vi "Vision Processing.vi"(4 "error in (no error)":errorcluster, 6 "CameraDevRef":T1) -> ()   [LabVIEW 2011]
uses:
  <vilib>/Rock Robotics/WPI/Camera/WPI_CameraDevRef.ctl
  Robot Global Data.vi
  <vilib>/vision/NI_Vision_Development_Module.lvlib
panel:
  in  "AntiDrift":dbl=-0.065
  in  "Y AbsolVal Difference":dbl=0.25
  in  "Default Shooter Speed Dump":dbl=0.4
  in  "Scale":dbl=0.85
  in  "Minimum Power":dbl=0.22
  out "Aspect Ratio":dbl[](array[numeric])
  out "Offset":dbl
  out "Raw Turret":dbl
  out "Target X Coord":dbl
  out "Target Distance":dbl
  out "Distance Array":dbl[](array[numeric])
  in  "Dead Band":dbl=0.09
  out "Number of Rectangles Visible":dbl
  out "Y Position Array":dbl[](array[numeric])
  out "X Position Array":dbl[](array[numeric])
  in  "View":bool
  out "Target Info":T2(array[cluster])
  in  "Area Size Limit":i32=444
  in  "Particle Count Limit":i32=8
  in  "Score Limits":T3={"Rect Coverage"=76.0, "Aspect Ratio"=40.0, "X Edge Strength"=40.0, "Y Edge Strength"=60.0}
  in  "Processing":enum32{"Color", "Intensity", "Intensity Open"}(tab)=enum."Intensity"
  in  "Luminance":i32=255
  in  "Saturation":i32=255
  in  "Hue":i32(knob)=65 scale=0.0..255.0
  in  "Margins":cluster{"Hue":i32, "Sat":i32, "Lum":i32}={"Hue"=20, "Sat"=27, "Lum"=30} {"Sat" scale=0.0..40.0; "Lum" scale=0.0..40.0; "Hue" scale=0.0..40.0}
  in  "Range":cluster{"Lower value":sgl, "Upper value":sgl}={"Lower value"=151.52174, "Upper value"=255.0} {"Lower value" scale=0.0..255.0; "Upper value" scale=0.0..255.0}
  in  "Range":cluster{"Lower value":sgl, "Upper value":sgl}={"Lower value"=123.804344, "Upper value"=255.0} {"Lower value" scale=0.0..255.0; "Upper value" scale=0.0..255.0}
  in  "View":bool
  out "Processed Image":T4(plugin-control)
  out "Original Image":T4(plugin-control)
  # "Instructions:\nProcessing the reflective tape that is illuminated by a ring light can be based\non color or light intensity.\nParticles within the image are scored by rectangle coverage, aspect ratio, and\nfor being hollow with a bold edge. A particle is considered a target if all scores\nare above the score limits. Particles can be annotated -- surrounded by\na rectangle and scores drawn to the left .\nTo control the number of particles being scored, use the count limit and the size\nlimit."
  # "(in)"
  # "To debug, Enable using the View button.\nFor color processing, you can click in the image to select the color for processing."
  # "Enable by clicking the View button.\nGreen scores are above the limit, orange are below. Inner/outer rect\nindicates all passed."
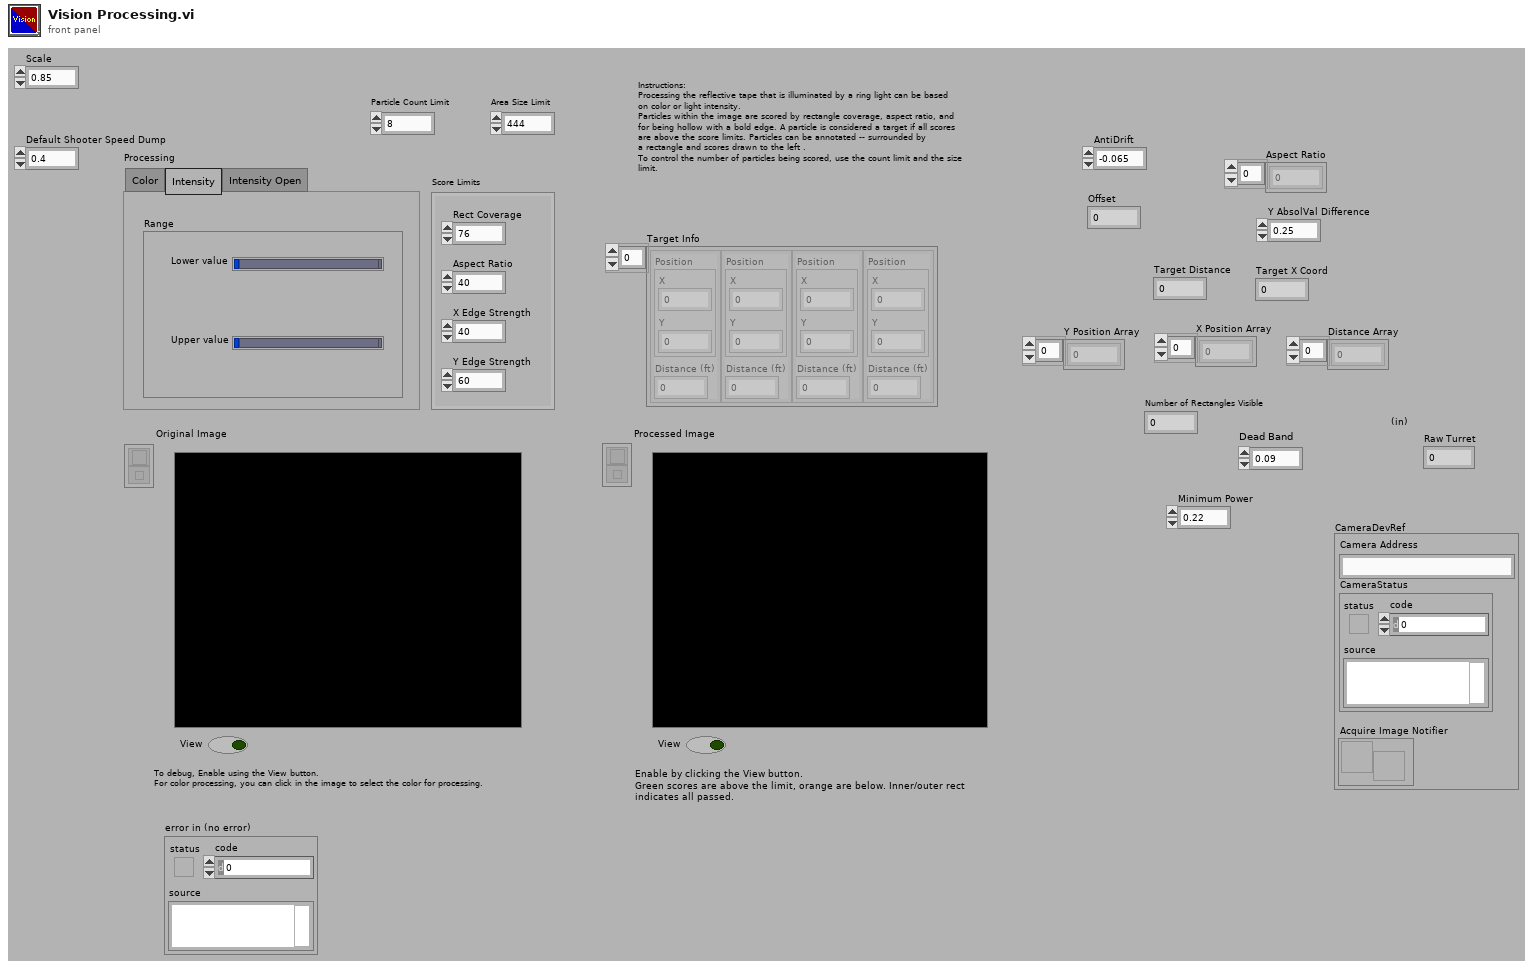
[diagram p1: front panel]
types:
  T1 = typedef "WPI_CameraDevRef.ctl" = cluster{"Camera Address":string, "CameraStatus":errorcluster, "Acquire Image Notifier":refnum<notifier>}
  T2 = cluster{"Position":cluster{"X":dbl, "Y":dbl}, "Distance (ft)":dbl}[]
  T3 = cluster{"Rect Coverage":dbl, "Aspect Ratio":dbl, "X Edge Strength":dbl, "Y Edge Strength":dbl}
  T4 = typedef "IMAQ Image.ctl" = refnum<image>
  T5 = typedef "Image Type" = u32
  T6 = enum32{"AutoM", "Close", "Dilate", "Erode", "Gradient", "Gradient out", "Gradient in", "Hit miss", "Open", "PClose", "POpen", "Thick", "Thin"}
  T7 = typedef "WPI_CameraImageSize.ctl" = enum16{"640x480", "320x240", "160x120"}
  T8 = cluster{"fps":i32, "compression":i32, "Image Size":T7}
  T9 = cluster{cluster{"Left":dbl, "Top":dbl, "Right":dbl, "Bottom":dbl}, dbl[]}[]
  T10 = cluster{"Left":dbl, "Top":dbl, "Right":dbl, "Bottom":dbl}
  T11 = cluster{"Target Center (-1 to 1)":cluster{"X":dbl, "Y":dbl}, "Distance (ft)":dbl}
  T12 = cluster{"Target Center (-1 to 1)":cluster{"X":dbl, "Y":dbl}, "Distance (ft)":dbl}[]
  T13 = typedef "WPI_JoystickDevRef.ctl" = cluster{"Device":T14}
  T14 = typedef "WPI_JoystickDeviceEnum.ctl" = enum16{"USB 1", "USB 2", "USB 3", "USB 4", "Kinect 1", "Kinect 2"}
  T15 = typedef "WPI_JoystickButtonState.ctl" = cluster{"Button 1":bool, "Button 2":bool, "Button 3":bool, "Button 4":bool, "Button 5":bool, "Button 6":bool, "Button 7":bool, "Button 8":bool, "Button 9":bool, "Button 10":bool, "Button 11":bool, "Button 12":bool}
  T16 = cluster{"axis 1 (x)":dbl, "axis 2 (y)":dbl, "axis 3 (throttle)":dbl, "axis 4":dbl, "axis 5":dbl, "axis 6":dbl}
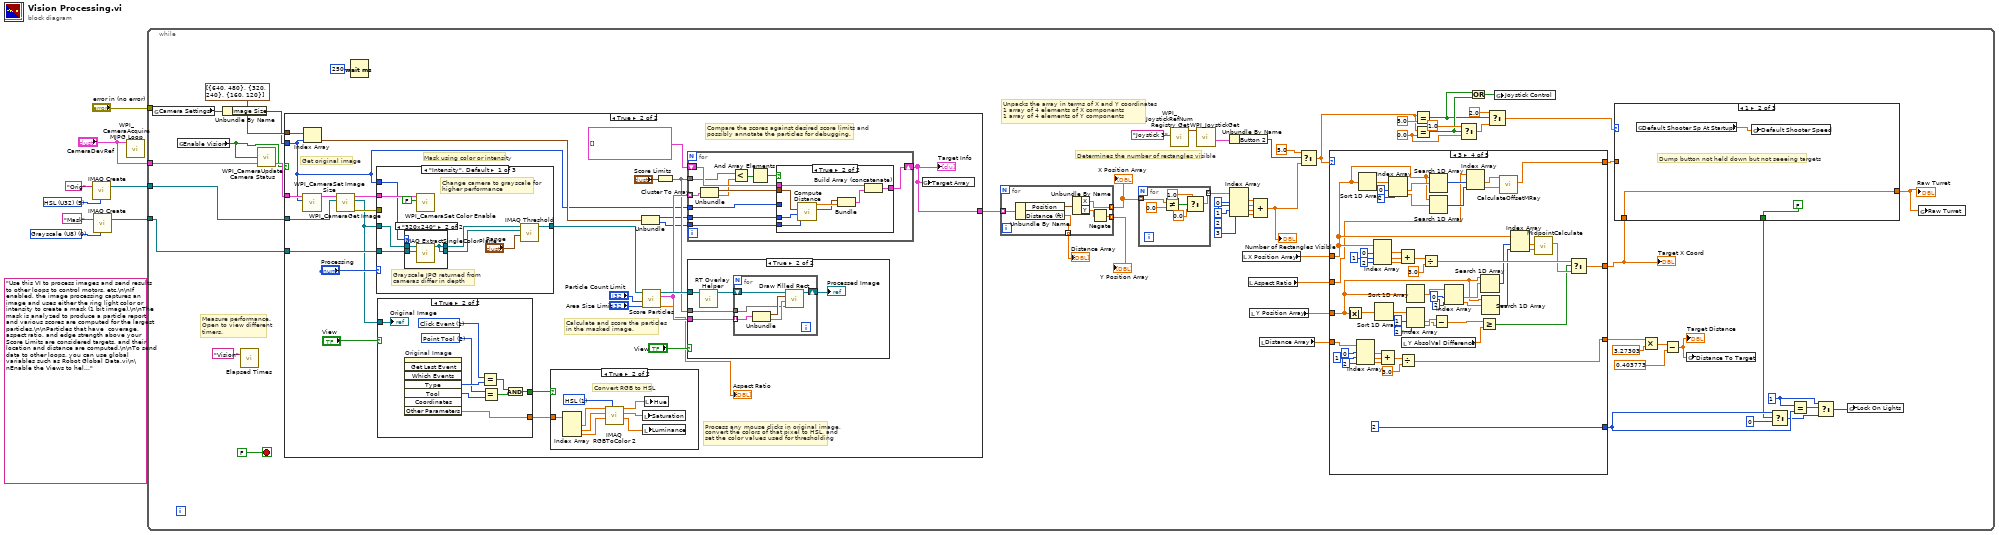
[diagram p0: block diagram]
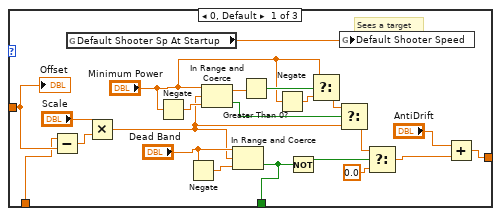
[diagram p2: hidden frame]
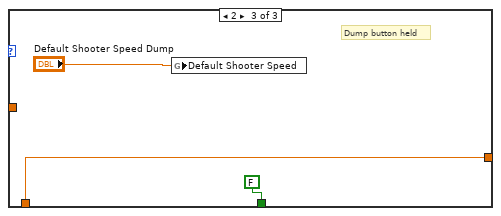
[diagram p3: hidden frame]
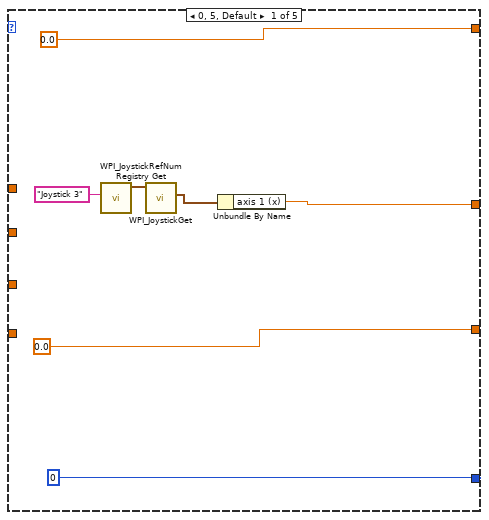
[diagram p4: hidden frame]
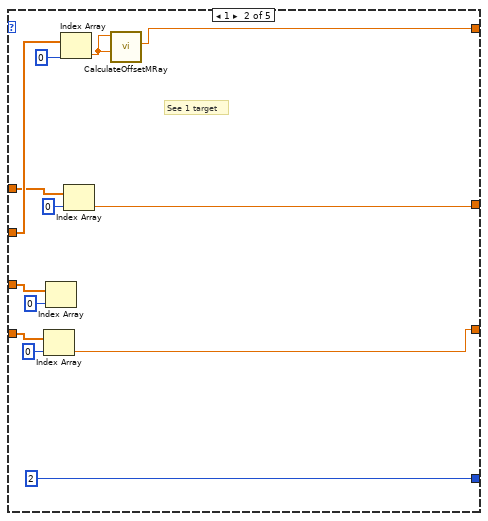
[diagram p5: hidden frame]
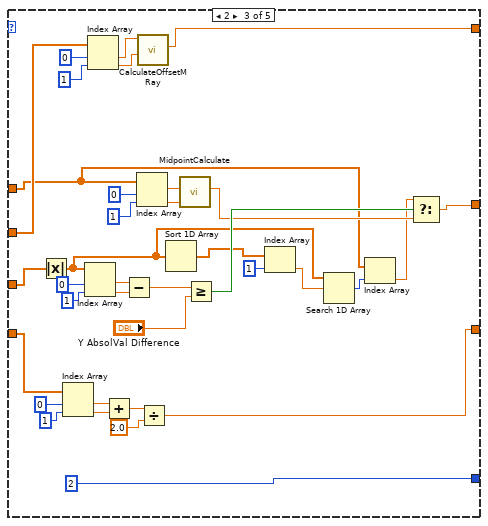
[diagram p6: hidden frame]
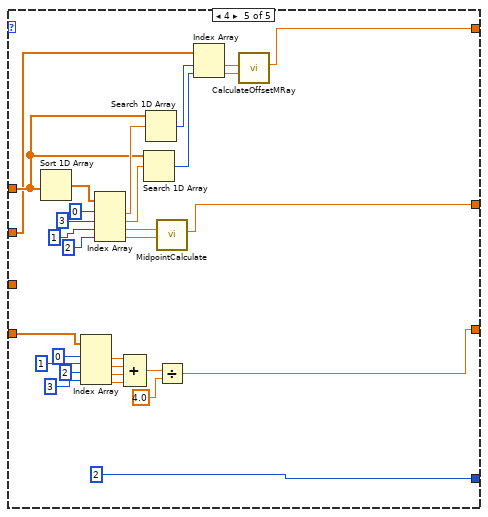
[diagram p7: hidden frame]
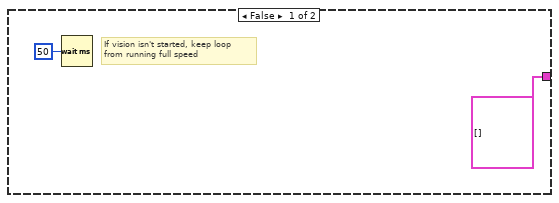
[diagram p8: hidden frame]
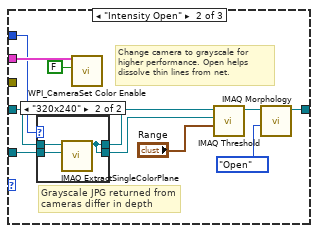
[diagram p11: hidden frame]
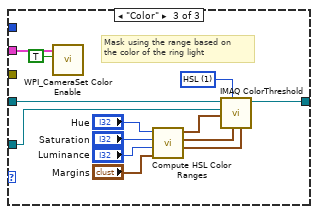
[diagram p13: hidden frame]
diagram:
  w3 = T5 0 items=["Grayscale (U8)", "Grayscale (I16)", "Grayscale (SGL)", "Complex (CSG)", "RGB (U32)", "HSL (U32)", "RGB (U64)", "Grayscale (U16)"] ("Image Type")
  (unwired) "Use this VI to process images and send results to other loops to control motors, etc.\n\nIf enabled, the image processing captures an image and uses either the ring light color or intensity to create a mask (1 bit image).\n\nThe mask is analyzed to produce a particle report and various scores are computed for the largest particles.\n\nParticles that have  coverage, aspect ratio, and edge strength above your Score Limits are considered targets, and their location and distance are computed.\n\nTo send data to other loops, you can use global variables such as Robot Global Data.vi\n\nEnable the Views to help debug color settings. Disable the View to speed up processing."
  w7 = T5 5 items=["Grayscale (U8)", "Grayscale (I16)", "Grayscale (SGL)", "Complex (CSG)", "RGB (U32)", "HSL (U32)", "RGB (U64)", "Grayscale (U16)"] ("Image Type")
  n1 = call "IMAQ Create"("Image Name"="Orig", "Image Type"=w7) -> ("New Image"=w6:T4)  [unwired: 2 in, 2 out]
  n2 = call "IMAQ Create"("Image Name"="Mask", "Image Type"=w3) -> ("New Image"=w1:T4)  [unwired: 2 in, 2 out]
  n3 = call <vilib>:"WPI_CameraAcquire MJPG Loop.vi"("CameraDevRef"="CameraDevRef") -> ()  [unwired: 11 in]
  n4 = while {
    tunnel: w6 -> [w66]
    tunnel: "CameraDevRef" -> [w65]
    tunnel: "error in (no error)" -> [_]
    tunnel: w1 -> [w61]
    stop <- FALSE stop-if-true
    w14 = 0.0 ("y")
    w31 = 1 ("y")
    # "Determines the number of rectangles visible"
    # "Unpacks the array in terms of X and Y coordinates\n1 array of 4 elements of X components\n1 array of 4 elements of Y components"
    # "Measure performance.\nOpen to view different\ntimers."
    n5 = global read "Robot Global Data.vi" "Camera Settings"() -> (w59:T8)
    n6 = global read "Robot Global Data.vi" "Enable Vision"() -> (w63:bool)
    n7 = Unbundle By Name(w59) -> ("Image Size"=w58:T7)
    n8 = call "Elapsed Times.vi"("Call Name"="Vision") -> ()  [unwired: 2 in, 1 out]
    n9 = call <vilib>:"WPI_CameraUpdate Camera Status.vi"("CameraDevRef In"=w65, "Enable Vision"=w63) -> ("CameraDevRef Out"=w64:T1)  [unwired: 3 in]
    n10 = case shown="True" w63 {
      tunnel: w66 -> [_ w266]
      tunnel: w64 -> [_ w262]
      tunnel: w61 -> [_ w253]
      tunnel: cluster{i32, i32}[] [{640, 480}, {320, 240}, {160, 120}] -> [_ w257]
      tunnel: w58 -> [_ w250]
      tunnel: [T2 [] w251] -> w57
      frame False {
        # "If vision isn't started, keep loop\nfrom running full speed"
        n11 = Wait (ms)(milliseconds to wait=u32 50) -> ()  [unwired: 1 out]
      }
      frame True {
        # "Compare the scores against desired score limits and\npossibly annotate the particles for debugging."
        # "Process any mouse clicks in original image,\nconvert the colors of that pixel to HSL, and\nset the color values used for thresholding"
        # "Calculate and score the particles\nin the masked image."
        # "Mask using color or intensity"
        # "Get original image"
        n12 = call <vilib>:"WPI_CameraSet Image Size.vi"("Image Size"=w250, "CameraDevRef"=w262) -> ("CameraDevRef Out"=w263:T1)  [unwired: 8 in, 1 out]
        n13 = Index Array(array=w257, index=w250) -> (element=w254:cluster{i32, i32})
        n14 = call <vilib>:"WPI_CameraGet Image.vi"("Image"=w266, "CameraDevRef"=w263) -> ("error out"=w264:errorcluster, "Image Out"=w252:T4, "CameraDevRef Out"=w265:T1)  [unwired: 7 in]
        n15 = case shown="\"Intensity\", Default" "Processing" {
          tunnel: w252 -> [w288 w300 w326]
          tunnel: [w291 w305 w325] -> w260
          tunnel: w265 -> [w289 w303 w316]
          tunnel: w264 -> [_ _ _]
          tunnel: w253 -> [w287 w301 w314]
          tunnel: w250 -> [w286 w302 _]
          frame "Intensity", Default {
            # "Grayscale JPG returned from\ncameras differ in depth"
            # "Change camera to grayscale for\nhigher performance"
            n16 = case shown="\"320x240\"" w286 {
              tunnel: w288 -> [w294 w297]
              tunnel: w287 -> [w293 w296]
              tunnel: [w294 w295] -> w285
              tunnel: [w293 w295] -> w284
              frame "640x480", Default {
              }
              frame "320x240" {
                n17 = call "IMAQ ExtractSingleColorPlane"("Image Dst"=w296, "Image Src"=w297) -> ("Image Dst Out"=w295:T4)  [unwired: 8 in, 1 out]
              }
            }
            n18 = call <vilib>:"WPI_CameraSet Color Enable.vi"("Color Enabled"=FALSE, "CameraDevRef"=w289) -> ()  [unwired: 8 in, 2 out]
            n19 = call "IMAQ Threshold"("Range"="Range", "Image Dst"=w284, "Image Src"=w285) -> ("Image Dst Out"=w291:T4)  [unwired: 3 in, 5 out]
          }
          frame "Intensity Open" {
            # "Grayscale JPG returned from\ncameras differ in depth"
            # "Change camera to grayscale for\nhigher performance. Open helps\ndissolve thin lines from net."
            n20 = case shown="\"320x240\"" w302 {
              tunnel: w300 -> [w310 w313]
              tunnel: w301 -> [w309 w312]
              tunnel: [w310 w311] -> w299
              tunnel: [w309 w311] -> w298
              frame "640x480", Default {
              }
              frame "320x240" {
                n21 = call "IMAQ ExtractSingleColorPlane"("Image Dst"=w312, "Image Src"=w313) -> ("Image Dst Out"=w311:T4)  [unwired: 8 in, 1 out]
              }
            }
            n22 = call <vilib>:"WPI_CameraSet Color Enable.vi"("Color Enabled"=FALSE, "CameraDevRef"=w303) -> ()  [unwired: 8 in, 2 out]
            n23 = call "IMAQ Threshold"("Range"="Range", "Image Dst"=w298, "Image Src"=w299) -> ("Image Dst Out"=w306:T4)  [unwired: 3 in, 5 out]
            n24 = call "IMAQ Morphology"("Operation"=T6."Open", "Image Src"=w306) -> ("Image Dst Out"=w305:T4)  [unwired: 8 in, 1 out]
          }
          frame "Color" {
            w324 = u16 1 items=["RGB", "HSL", "HSV", "HSI"] ("Color Mode")
            # "Mask using the range based on\nthe color of the ring light"
            n25 = call <vilib>:"WPI_CameraSet Color Enable.vi"("Color Enabled"=TRUE, "CameraDevRef"=w316) -> ()  [unwired: 8 in, 2 out]
            n26 = call "Compute HSL Color Ranges.vi"("Margins"="Margins", "Luminance"="Luminance", "Saturation"="Saturation", "Hue"="Hue") -> ("Lum Range"=w321:cluster{i32, i32}, "Sat Range"=w322:cluster{i32, i32}, "Hue Range"=w323:cluster{i32, i32})  [unwired: 5 in]
            n27 = call "IMAQ ColorThreshold"("Blue or Luma or Val or Inten Range"=w321, "Green or Sat Range"=w322, "Color Mode"=w324, "Red or Hue Range"=w323, "Image Dst"=w314, "Image Src"=w326) -> ("Image Dst Out"=w325:T4)  [unwired: 4 in, 1 out]
          }
        }
        n28 = case shown="True" "View" {
          tunnel: w252 -> [_ w346]
          tunnel: [_ w341] -> w259
          tunnel: [_ w338] -> w258
          frame False {
          }
          frame True {
            w339 = 2 items=["None", "Selection Tool", "Point Tool", "Line Tool", "Rectangle Tool", "Oval Tool", "Polygon Tool", "ClosedFreehandTool", "Annulus Tool", "Rotated Rectangle Tool", "Zoom Tool", "Pan Tool", "Polyline Tool", "Freehand Tool"] ("Tool")
            w340 = 1 items=["No Event"=0, "Click Event"=1, "Draw Event"=2, "Size Event"=4, "Scroll Event"=5, "Double Click Event"=8] ("Type")
            n29 = invoke on="Original Image" class="ImageControl" method="Get Last Event"() -> ("Type"=w342:i32, "Tool"=w345:i32, "Other Parameters"=w338:sgl[])  [unwired: 8 in, 5 out]
            n30 = Equal?(x=w340, y=w342) -> (x = y?=w343:bool)
            n31 = Equal?(x=w339, y=w345) -> (x = y?=w344:bool)
            n32 = And(x=w343, y=w344) -> (x .and. y?=w341:bool)
            "Original Image" <- w346
          }
        }
        n33 = case shown="True" w259 {
          tunnel: w258 -> [_ w283]
          frame False {
          }
          frame True {
            w282 = u16 1 items=["RGB", "HSL", "HSV", "HSI", "CIE L*a*b*", "CIE XYZ"] ("Color Mode")
            # "Convert RGB to HSL"
            n34 = Index Array(array=w283) -> (element #1=w281:sgl, element #2=w279:sgl, element #3=w277:sgl)  [unwired: 3 in]
            n35 = call "IMAQ RGBToColor 2"("Color Mode"=w282, "Blue value"=w277, "Green value"=w279, "Red value"=w281) -> ("Blue or Luma or Val or Inten or Z or b*value"=w276:dbl, "Green or Sat or Y or a* value"=w278:dbl, "Red or Hue or X or L* value"=w280:dbl)  [unwired: 4 in, 1 out]
            n36 = local write "Saturation"(w278) -> ()
            n37 = local write "Luminance"(w276) -> ()
            n38 = local write "Hue"(w280) -> ()
          }
        }
        n39 = Unbundle(w254) -> (w256:i32, w255:i32)
        n40 = call "Score Particles.vi"("Area Size Limit"="Area Size Limit", "Particle Count Limit"="Particle Count Limit", "Image Refnum in"=w260) -> ("Aspect Ratio"=→"Aspect Ratio":dbl[], "Scored Particle Info"=w271:T9, "Image Refnum out"=w274:T4)  [unwired: 6 in]
        n41 = Cluster To Array(cluster="Score Limits") -> (array=w269:dbl[])
        n42 = for {
          shift-right: [w356] -> w251
          shift-left: T2 [] -> [w357]
          tunnel: w256 -> [w355]
          tunnel: w271 -> [w353] mode=indexing
          tunnel: w269 -> [w348]
          tunnel: w250 -> [w352]
          tunnel: w255 -> [w347]
          n43 = Unbundle(w353) -> (w354:T10, w349:dbl[])
          n44 = Less?(x=w348, y=w349) -> (x < y?=w351:bool[])
          n45 = And Array Elements(Boolean array=w351) -> (logical AND=w350:bool)
          n46 = case shown="True" w350 {
            tunnel: w357 -> [w358 w366]
            tunnel: [w358 w365] -> w356
            tunnel: w354 -> [_ w361]
            tunnel: w355 -> [_ w363]
            tunnel: w352 -> [_ _]
            tunnel: w347 -> [_ w360]
            frame False {
            }
            frame True {
              n47 = call "Compute Distance.vi"("Y Image Resolution"=w360, "X Image Resolution"=w363, "Bounding Box"=w361) -> ("Target Center (-1 to 1)"=w359:cluster{"X":dbl, "Y":dbl}, "Distance (ft)"=w362:dbl)  [unwired: 7 in]
              n48 = Bundle("Target Center (-1 to 1)"=w359, "Distance (ft)"=w362) -> (w364:T11)  [unwired: 1 in]
              n49 = Build Array (concatenate)(w366, w364) -> (w365:T12)
            }
          }
        }
        "Target Info" <- w251
        n50 = case shown="True" "View" {
          tunnel: w274 -> [_ w328]
          tunnel: w271 -> [_ w330]
          tunnel: w269 -> [_ w329]
          frame False {
          }
          frame True {
            n51 = call "RT Overlay Helper.vi"("Refnum in"=w328) -> ("Refnum out"=w331:T4)  [unwired: 10 in]
            n52 = for {
              shift-right: [w336] -> w327
              shift-left: w331 -> [w337]
              tunnel: w330 -> [w333] mode=indexing
              tunnel: w329 -> [w332]
              n53 = Unbundle(w333) -> (w334:T10, w335:dbl[])
              n54 = call "Draw Filled Rect.vi"("Limits"=w332, "Scores"=w335, "Bounding Box"=w334, "image in"=w337) -> ("image out"=w336:T4)  [unwired: 7 in]
            }
            "Processed Image" <- w327
          }
        }
        n55 = global write "Robot Global Data.vi" "Target Array"(w251) -> ()
      }
    }
    n56 = Wait (ms)(milliseconds to wait=u32 250) -> ()  [unwired: 1 out]
    n57 = for {
      tunnel: [w244] -> w37 mode=indexing
      tunnel: [w245] -> w47 mode=indexing
      tunnel: w57 -> [w242] mode=indexing
      tunnel: [w241] -> w49 mode=indexing
      n58 = Unbundle By Name(w242) -> ("Position"=w246:cluster{"X":dbl, "Y":dbl}, "Distance (ft)"=w241:dbl)
      n59 = Unbundle By Name(w246) -> ("X"=w245:dbl, "Y"=w243:dbl)
      n60 = Negate(x=w243) -> (-x=w244:dbl)
    }
    "X Position Array" <- w47
    "Y Position Array" <- w37
    "Distance Array" <- w49
    n61 = for {
      tunnel: w47 -> [w100] mode=indexing
      tunnel: [w96] -> w46 mode=indexing
      n62 = Not Equal?(x=w100, y=0.0) -> (x != y?=w99:bool)
      n63 = Select(t=1.0, s=w99, f=0.0) -> (s? t:f=w96:dbl)
    }
    n64 = call <vilib>:"WPI_JoystickRefNum Registry Get.vi"("refnum name"="Joystick 3") -> ("JoystickDevRef"=w36:T13)  [unwired: 9 in, 1 out]
    n65 = call <vilib>:"WPI_JoystickGet.vi"("JoystickDevRef"=w36) -> ("Buttons"=w34:T15)  [unwired: 4 in, 2 out]
    n66 = Unbundle By Name(w34) -> ("Button 2"=w33:bool)
    n67 = Index Array(array=w46, index #1=0 ("index"), index #2=1 ("index"), index #3=2 ("index"), index #4=3 ("index")) -> (element #1=w44:dbl, element #2=w45:dbl, element #3=w43:dbl, element #4=w42:dbl)
    n68 = local read "X Position Array"() -> (w48:dbl[])
    n69 = local read "Aspect Ratio"() -> (w26:dbl[])
    n70 = local read "Y Position Array"() -> (w50:dbl[])
    n71 = Compound Arithmetic op=ADD(w44, w45, w43, w42) -> (w27:dbl)
    "Number of Rectangles Visible" <- w27
    n72 = local read "Distance Array"() -> (w51:dbl[])
    n73 = Select(t=5.0, s=w33, f=w27) -> (s? t:f=w13:dbl)
    n74 = case shown="3" w13 {
      tunnel: w48 -> [_ w116 w123 w165 w216]
      tunnel: [w104 w115 w147 w199 w239] -> w24
      tunnel: w50 -> [_ w113 w146 w177 _]
      tunnel: w51 -> [_ w111 w135 w208 w236]
      tunnel: [0 2 2 2 2] -> w30
      tunnel: [0.0 ("Offset") w118 w152 w158 w225] -> w25
      tunnel: w26 -> [_ w121 w155 w161 w211]
      tunnel: [0.0 w110 w130 w201 w226] -> w19
      frame 0, 5, Default {
        n75 = call <vilib>:"WPI_JoystickRefNum Registry Get.vi"("refnum name"="Joystick 3") -> ("JoystickDevRef"=w103:T13)  [unwired: 9 in, 1 out]
        n76 = call <vilib>:"WPI_JoystickGet.vi"("JoystickDevRef"=w103) -> ("Axes"=w105:T16)  [unwired: 4 in, 2 out]
        n77 = Unbundle By Name(w105) -> ("axis 1 (x)"=w104:dbl)
      }
      frame 1 {
        # "See 1 target"
        n78 = Index Array(array=w111, index=0) -> (element=w110:dbl)
        n79 = Index Array(array=w113, index=0) -> ()  [unwired: 1 out]
        n80 = Index Array(array=w121, index=0) -> (element=w119:dbl)
        n81 = Index Array(array=w116, index=0) -> (element=w115:dbl)
        n82 = call "CalculateOffsetMRay.vi"("AR2"=w119, "AR1"=w119) -> ("Offset"=w118:dbl)  [unwired: 9 in]
      }
      frame 2 {
        n83 = Absolute Value(x=w146) -> (abs(x)=w126:dbl[])
        n84 = Index Array(array=w135, index #1=0 ("index"), index #2=1 ("index")) -> (element #1=w133:dbl, element #2=w134:dbl)
        n85 = Index Array(array=w126, index #1=0 ("index"), index #2=1 ("index")) -> (element #1=w142:dbl, element #2=w143:dbl)
        n86 = Index Array(array=w155, index #1=0 ("index"), index #2=1 ("index")) -> (element #1=w154:dbl, element #2=w153:dbl)
        n87 = Add(x=w133, y=w134) -> (x+y=w132:dbl)
        n88 = Subtract(x=w142, y=w143) -> (x-y=w141:dbl)
        n89 = Index Array(array=w123, index #1=0 ("index"), index #2=1 ("index")) -> (element #1=w148:dbl, element #2=w149:dbl)
        n90 = call "CalculateOffsetMRay.vi"("AR2"=w153, "AR1"=w154) -> ("Offset"=w152:dbl)  [unwired: 9 in]
        n91 = Divide(x=w132, y=2.0) -> (x/y=w130:dbl)
        n92 = Sort 1D Array(array=w126) -> (sorted array=w128:dbl[])
        n93 = call "MidpointCalculate.vi"("X2"=w149, "X1"=w148) -> ("Midpoint"=w138:dbl)  [unwired: 9 in]
        n94 = Greater Or Equal?(x=w141, y="Y AbsolVal Difference") -> (x >= y?=w139:bool)
        n95 = Index Array(array=w128, index=1) -> (element=w125:dbl)
        n96 = Search 1D Array(1D array=w126, element=w125) -> (index of element=w124:i32)  [unwired: 1 in]
        n97 = Index Array(array=w123, index=w124) -> (element=w122:dbl)
        n98 = Select(t=w122, s=w139, f=w138) -> (s? t:f=w147:dbl)
      }
      frame 3 {
        n99 = Absolute Value(x=w177) -> (abs(x)=w198:dbl[])
        n100 = Index Array(array=w208, index #1=0 ("index"), index #2=1 ("index"), index #3=2 ("index")) -> (element #1=w204:dbl, element #2=w205:dbl, element #3=w206:dbl)
        n101 = Sort 1D Array(array=w165) -> (sorted array=w169:dbl[])
        n102 = Index Array(array=w165, index #1=0 ("index"), index #2=1 ("index"), index #3=2 ("index")) -> (element #1=w186:dbl, element #2=w188:dbl, element #3=w187:dbl)
        n103 = Sort 1D Array(array=w198) -> (sorted array=w182:dbl[])
        n104 = Compound Arithmetic op=ADD(w204, w205, w206) -> (w203:dbl)
        n105 = Index Array(array=w169, index #1=0 ("index"), index #2=2 ("index")) -> (element #1=w166:dbl, element #2=w164:dbl)
        n106 = Divide(x=w203, y=3.0) -> (x/y=w201:dbl)
        n107 = Compound Arithmetic op=ADD(w186, w188, w187) -> (w185:dbl)
        n108 = local read "Y AbsolVal Difference"() -> (w192:dbl)
        n109 = Sort 1D Array(array=w177) -> (sorted array=w181:dbl[])
        n110 = Index Array(array=w182, index #1=1 ("index"), index #2=2 ("index")) -> (element #1=w194:dbl, element #2=w195:dbl)
        n111 = Divide(x=w185, y=3.0) -> (x/y=w183:dbl)
        n112 = Search 1D Array(1D array=w165, element=w166) -> (index of element=w163:i32)  [unwired: 1 in]
        n113 = Search 1D Array(1D array=w165, element=w164) -> (index of element=w162:i32)  [unwired: 1 in]
        n114 = Subtract(x=w195, y=w194) -> (x-y=w193:dbl)
        n115 = Index Array(array=w181, index #1=0 ("index"), index #2=2 ("index")) -> (element #1=w178:dbl, element #2=w176:dbl)
        n116 = Index Array(array=w161, index #1=w163, index #2=w162) -> (element #1=w160:dbl, element #2=w159:dbl)
        n117 = Greater Or Equal?(x=w193, y=w192) -> (x >= y?=w170:bool)
        n118 = Search 1D Array(1D array=w177, element=w178) -> (index of element=w175:i32)  [unwired: 1 in]
        n119 = Search 1D Array(1D array=w177, element=w176) -> (index of element=w174:i32)  [unwired: 1 in]
        n120 = call "CalculateOffsetMRay.vi"("AR2"=w159, "AR1"=w160) -> ("Offset"=w158:dbl)  [unwired: 9 in]
        n121 = Index Array(array=w165, index #1=w175, index #2=w174) -> (element #1=w172:dbl, element #2=w173:dbl)
        n122 = call "MidpointCalculate.vi"("X2"=w173, "X1"=w172) -> ("Midpoint"=w171:dbl)  [unwired: 9 in]
        n123 = Select(t=w183, s=w170, f=w171) -> (s? t:f=w199:dbl)
      }
      frame 4 {
        n124 = Sort 1D Array(array=w216) -> (sorted array=w240:dbl[])
        n125 = Index Array(array=w236, index #1=0 ("index"), index #2=1 ("index"), index #3=2 ("index"), index #4=3 ("index")) -> (element #1=w233:dbl, element #2=w232:dbl, element #3=w231:dbl, element #4=w230:dbl)
        n126 = Index Array(array=w240, index #1=0 ("index"), index #2=3 ("index"), index #3=1 ("index"), index #4=2 ("index")) -> (element #1=w217:dbl, element #2=w218:dbl, element #3=w224:dbl, element #4=w223:dbl)
        n127 = Compound Arithmetic op=ADD(w233, w232, w231, w230) -> (w229:dbl)
        n128 = Search 1D Array(1D array=w216, element=w218) -> (index of element=w213:i32)  [unwired: 1 in]
        n129 = Search 1D Array(1D array=w216, element=w217) -> (index of element=w212:i32)  [unwired: 1 in]
        n130 = call "MidpointCalculate.vi"("X2"=w223, "X1"=w224) -> ("Midpoint"=w239:dbl)  [unwired: 9 in]
        n131 = Divide(x=w229, y=4.0) -> (x/y=w226:dbl)
        n132 = Index Array(array=w211, index #1=w212, index #2=w213) -> (element #1=w215:dbl, element #2=w214:dbl)
        n133 = call "CalculateOffsetMRay.vi"("AR2"=w214, "AR1"=w215) -> ("Offset"=w225:dbl)  [unwired: 9 in]
      }
    }
    "Target X Coord" <- w24
    n134 = Equal?(x=w13, y=5.0) -> (x = y?=w11:bool)
    n135 = Equal?(x=w13, y=w14) -> (x = y?=w12:bool)
    n136 = Select(t=1.0, s=w12, f=w14) -> (s? t:f=w17:dbl)
    n137 = Or(x=w11, y=w12) -> (x .or. y?=w10:bool)
    n138 = Select(t=2.0, s=w11, f=w17) -> (s? t:f=w9:dbl)
    n139 = global write "Robot Global Data.vi" "Joystick Control"(w10) -> ()
    n140 = case shown="1" w9 {
      tunnel: w25 -> [w88 _ _]
      tunnel: w24 -> [w87 w92 w95]
      tunnel: [w70 w92 w95] -> w55
      tunnel: [w73 FALSE FALSE] -> w23
      frame 0, Default {
        # "Sees a target"
        n141 = Subtract(x=w87, y=w88) -> (x-y=w85:dbl)
        n142 = global read "Robot Global Data.vi" "Default Shooter Sp At Startup"() -> (w68:dbl)
        n143 = Multiply(x="Scale", y=w85) -> (x*y=w76:dbl)
        n144 = Negate(x="Minimum Power") -> (-x=w83:dbl)
        n145 = Negate(x="Dead Band") -> (-x=w89:dbl)
        n146 = In Range and Coerce(upper limit="Minimum Power", x=w76, lower limit=w83) -> (coerced(x)=w79:dbl, In Range?=w80:bool)
        n147 = In Range and Coerce(upper limit="Dead Band", x=w76, lower limit=w89) -> (In Range?=w73:bool)  [unwired: 1 out]
        n148 = Greater Than 0?(x=w79) -> (x > 0?=w78:bool)
        n149 = Negate(x="Minimum Power") -> (-x=w75:dbl)
        n150 = Not(x=w73) -> (.not. x?=w74:bool)
        n151 = Select(t="Minimum Power", s=w78, f=w75) -> (s? t:f=w77:dbl)
        n152 = Select(t=w77, s=w80, f=w76) -> (s? t:f=w81:dbl)
        n153 = global write "Robot Global Data.vi" "Default Shooter Speed"(w68) -> ()
        n154 = Select(t=w81, s=w74, f=0.0) -> (s? t:f=w71:dbl)
        n155 = Add(x="AntiDrift", y=w71) -> (x+y=w70:dbl)
        "Offset" <- w88
      }
      frame 1 {
        # "Dump button not held down but not seeeing targets"
        n156 = global read "Robot Global Data.vi" "Default Shooter Sp At Startup"() -> (w90:dbl)
        n157 = global write "Robot Global Data.vi" "Default Shooter Speed"(w90) -> ()
      }
      frame 2 {
        # "Dump button held"
        n158 = global write "Robot Global Data.vi" "Default Shooter Speed"("Default Shooter Speed Dump") -> ()
      }
    }
    "Raw Turret" <- w55
    n159 = Multiply(x=w19, y=3.27303) -> (x*y=w22:dbl)
    n160 = Subtract(x=w22, y=0.403773) -> (x-y=w53:dbl)
    "Target Distance" <- w53
    n161 = global write "Robot Global Data.vi" "Distance To Target"(w53) -> ()
    n162 = Select(t=w30, s=w23, f=0) -> (s? t:f=w28:i32)
    n163 = Equal?(x=w31, y=w30) -> (x = y?=w32:bool)
    n164 = Select(t=w31, s=w32, f=w28) -> (s? t:f=w54:i32)
    n165 = global write "Robot Global Data.vi" "Lock On Lights"(w54) -> ()
    n166 = global write "Robot Global Data.vi" "Raw Turret"(w55) -> ()
  }
